vi "Encode Variant 2 String.vi"(8 "error in":errorcluster, 11 "Variant":variant) -> (0 "error out":errorcluster, 3 "String Output":string)   [LabVIEW 2022 SP3]
doc: "Encodes a Variant in a string by encoding the array of types as well.\n\n(c) 2022 Scott Hannahs <sth@magnet.fsu.edu>\nVersion 1 9/23/2022"
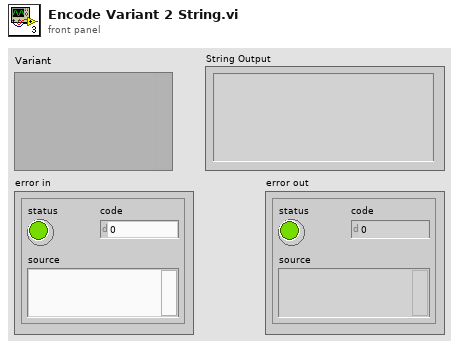
[diagram p1: front panel]
types:
  T1 = enum16{"big-endian, network order", "native, host order", "little-endian"}
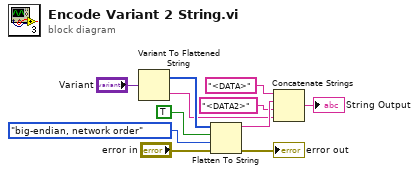
[diagram p0: block diagram]
diagram:
  n1 = Variant To Flattened String(Variant="Variant") -> (data string=w8:string, 1:w10:i16[])
  n2 = Flatten To String(anything=w10, prepend array or string size? (T)=TRUE, byte order (0:big-endian, network order)=T1."big-endian, network order", error in (no error)="error in") -> (data string=w9:string, error out=→"error out":errorcluster)  [unwired: 1 out]
  n3 = Concatenate Strings("<DATA>" ("string"), w9, "<DATA2>" ("string"), w8) -> (→"String Output":string)
